vi "Next.vi"(8 "error in (no error)":errorcluster, 11 "Steps in":refnum<class "Steps.lvclass">) -> (0 "error out":errorcluster, 1 "Step Number":i32, 2 "Reached End?":bool, 3 "Steps out":refnum<class "Steps.lvclass">)   [LabVIEW 2015, in "Steps.lvclass"]
doc: "This method moves the active tab to the next one that is currently active.\n\n<b> </b> <b> </b>\n©2016 Q Software Innovations, LLC (QSI)\nwritten by Quentin Alldredge\nproduced in LabVIEW 2015\n\nsupport@qsoftwareinnovations.com\nwww.qsoftwareinnovations.com\n\nAll rights reserved.\n\nRedistribution and use in source and binary forms, with or without modification, are permitted provided that the following conditions are met:\n\n * Redistributions of source code must retain the above copyright notice, this list of conditions and the following disclaimer.\n * Redistributions in binary form must reproduce the above copyright notice, this list of conditions and the following disclaimer in the documentation and/or other materials provided with the distribution.\n * Neither the name of Q Software Innovations, LLC. nor the names of its contributors may be used to endorse or promote products derived from this software without specific prior written permission.\n\nTHIS SOFTWARE IS PROVIDED BY THE COPYRIGHT HOLDERS AND CONTRIBUTORS \"AS IS\" AND ANY EXPRESS OR IMPLIED WARRANTIES, INCLUDING, BUT NOT LIMITED TO, THE IMPLIED WARRANTIES OF MERCHANTABILITY AND FITNESS FOR A PARTICULAR PURPOSE ARE DISCLAIMED. IN NO EVENT SHALL THE COPYRIGHT OWNER OR CONTRIBUTORS BE LIABLE FOR ANY DIRECT, INDIRECT, INCIDENTAL, SPECIAL, EXEMPLARY, OR CONSEQUENTIAL DAMAGES (INCLUDING, BUT NOT LIMITED TO, PROCUREMENT OF SUBSTITUTE GOODS OR SERVICES; LOSS OF USE, DATA, OR PROFITS; OR BUSINESS INTERRUPTION) HOWEVER CAUSED AND ON ANY THEORY OF LIABILITY, WHETHER IN CONTRACT, STRICT LIABILITY, OR TORT (INCLUDING NEGLIGENCE OR OTHERWISE) ARISING IN ANY WAY OUT OF THE USE OF THIS SOFTWARE, EVEN IF ADVISED OF THE POSSIBILITY OF SUCH DAMAGE."
uses:
  Steps.lvclass
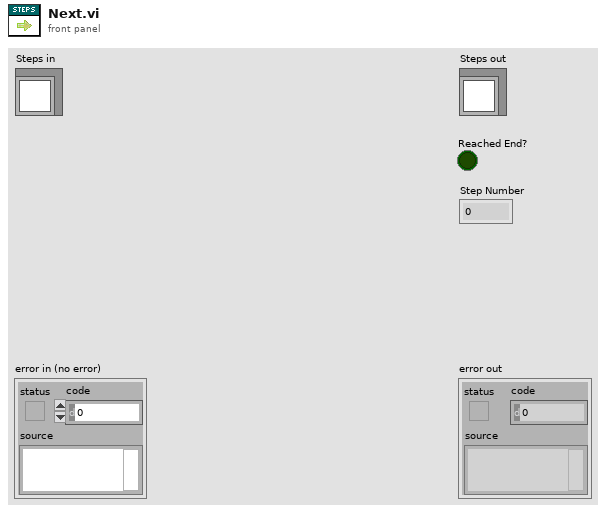
[diagram p1: front panel]
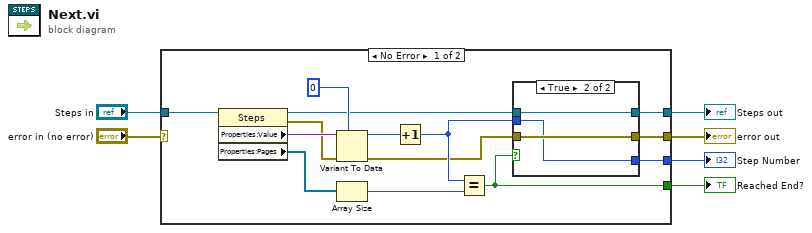
[diagram p0: block diagram]
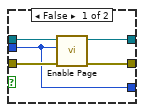
[diagram p2: hidden frame]
diagram:
  n1 = case shown="No Error" "error in (no error)" {
    selector: "error in (no error)" -> [_ w30]
    tunnel: [w8 w30] -> w5
    tunnel: [w15 w29] -> w3
    tunnel: "Steps in" -> [w20 w29]
    tunnel: [w10 _] -> w2
    tunnel: [w7 _] -> w1
    frame No Error {
      n2 = property class="Steps"(reference=w20) -> (reference out=w16:refnum<class "Steps.lvclass">, error out=w11:errorcluster, "Properties:Value"=w19:variant, "Properties:Pages"=w17:refnum<vi>[])  [unwired: 1 in]
      n3 = Variant To Data(error in=w11, type=0, Variant=w19) -> (data=w14:i32, error out=w9:errorcluster)
      n4 = Array Size(array=w17) -> (size(s)=w12:i32)
      n5 = Increment(x=w14) -> (x+1=w13:i32)
      n6 = Equal?(x=w13, y=w12) -> (x = y?=w10:bool)
      n7 = case shown="True" w10 {
        tunnel: w16 -> [w25 w28]
        tunnel: [w24 w28] -> w15
        tunnel: w13 -> [w21 w26]
        tunnel: w9 -> [w23 w27]
        tunnel: [w22 w27] -> w8
        tunnel: [w21 w26] -> w7
        frame False {
          n8 = call "Enable Page.vi"("error in (no error)"=w23, "Page Index"=w21, "Steps in"=w25) -> ("error out"=w22:errorcluster, "Steps out"=w24:refnum<class "Steps.lvclass">)  [unwired: 7 in]
        }
        frame True {
        }
      }
    }
    frame Error {
    }
  }
  "error out" <- w5
  "Steps out" <- w3
  "Reached End?" <- w2
  "Step Number" <- w1
